vi "Get Available Software extended.vi"(8 "error in (no error)":errorcluster, 10 "Item Types (all visible)":T3 items=["all visible", "all including hidden", "standard only", "startup only"], 11 "Session in":refnum<k21>) -> (0 "error out":errorcluster, 2 "Software Components":T1[](array[typedef]) {"Visibility Type" items=["standard", "hidden", "system", "unknown", "startup", "image"]}, 3 "Session out":refnum<k21>)   [LabVIEW 2012, in "nisyscfg.lvlib"]
uses:
  <vilib>/nisyscfg/nisyscfg.lvlib
  <vilib>/nisyscfg/Component Types.ctl
  <vilib>/nisyscfg/Software Extended.ctl
  <vilib>/nisyscfg/Component Type.ctl
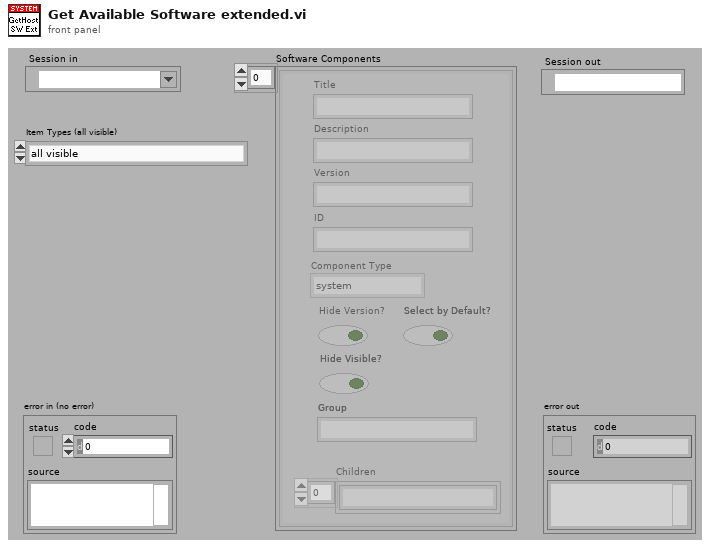
[diagram p1: front panel]
types:
  T1 = typedef "nisyscfg.lvlib/Software Extended.ctl" = cluster{"Description":string, "ID":string, "Version":string, "Title":string, "Visibility Type":T2, "Hide Version?":bool, "Children":string[], "Select by Default?":bool, "Hide Visible?":bool, "Group":string}
  T2 = typedef "nisyscfg.lvlib/Component Type.ctl" = u32
  T3 = typedef "nisyscfg.lvlib/Component Types.ctl" = u32
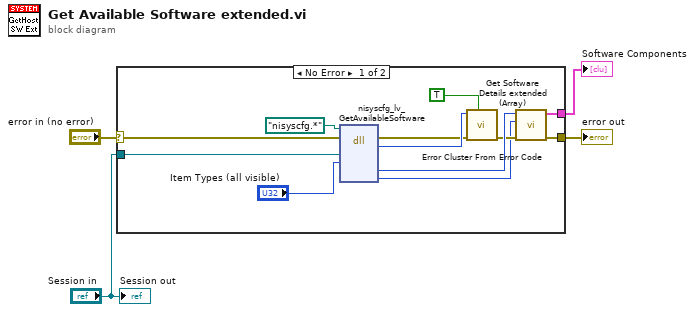
[diagram p0: block diagram]
diagram:
  n1 = case shown="No Error" "error in (no error)" {
    selector: "error in (no error)" -> [w14 w17]
    tunnel: [w7 w17] -> w4
    tunnel: "Session in" -> [w13 _]
    tunnel: [w8 _] -> w2
    frame No Error {
      n2 = dll-call lib="nisyscfg.*" fn="nisyscfg_lv_GetAvailableSoftware" label="GetAvailableSoftware"(path in=path "nisyscfg.*", error in=w14, "system"=w13, "includeTypes"="Item Types (all visible)") -> (error out=w15:errorcluster, "result"=w16:i32, "components"=w10:u64, "numComponents"=w6:i32)  [unwired: 5 in, 1 out]
      n3 = call <vilib>:"Error Cluster From Error Code.vi"("show call chain? (False)"=TRUE, "error in (no error)"=w15, "error code (0)"=w16) -> ("error out"=w9:errorcluster)  [unwired: 6 in]
      n4 = call <vilib>:"Get Software Details extended (Array).vi"("error in (no error)"=w9, "Number of Elements"=w6, "Enumerator in"=w10) -> ("error out"=w7:errorcluster, "Software Components"=w8:T1[])  [unwired: 7 in]
    }
    frame Error {
    }
  }
  "error out" <- w4
  "Software Components" <- w2
  "Session out" <- "Session in"
